vi "M1 Titanium Metal Properties.vi"(6 "m-nm M1":dbl, 9 "Metal 1 (Ti)":dbl, 10 "Energy (Heat; I^2R)":dbl, 11 "NS Base Area":dbl) -> (1 "Volume M1":dbl, 2 "Mass M1":dbl, 3 "Delta Temp Change M1":dbl, 4 "M1 Thickness":dbl, 5 "M1 Specfic Heat Capacity":dbl, 7 "M1 Density":dbl)   [LabVIEW 2020]
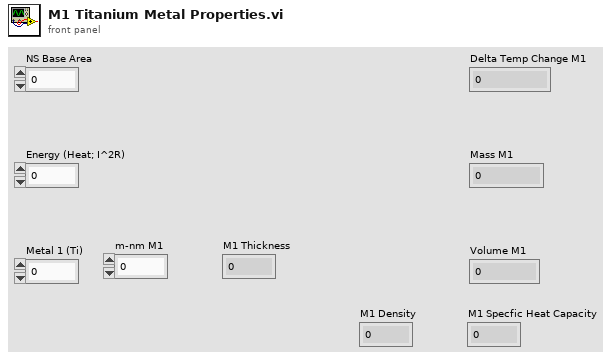
[diagram p1: front panel]
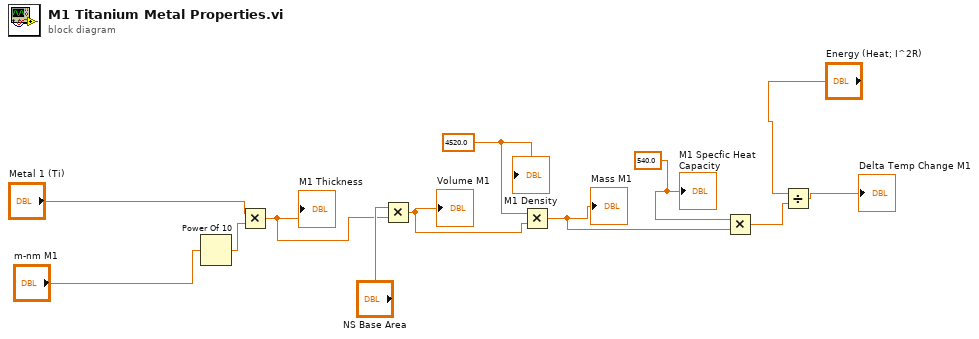
[diagram p0: block diagram]
diagram:
  w9 = 540.0 ("Silicon Specfic Heat Capacity 3")
  w5 = 4520.0 ("Silicon Density 3")
  n1 = Power Of 10(x="m-nm M1") -> (10^x=w1:dbl)
  n2 = Multiply(x="Metal 1 (Ti)", y=w1) -> (x*y=w4:dbl)
  "M1 Thickness" <- w4
  n3 = Multiply(x="NS Base Area", y=w4) -> (x*y=w6:dbl)
  "Volume M1" <- w6
  n4 = Multiply(x=w5, y=w6) -> (x*y=w8:dbl)
  "Mass M1" <- w8
  n5 = Multiply(x=w9, y=w8) -> (x*y=w11:dbl)
  n6 = Divide(x="Energy (Heat; I^2R)", y=w11) -> (x/y=→"Delta Temp Change M1":dbl)
  "M1 Density" <- w5
  "M1 Specfic Heat Capacity" <- w9
